vi "PH_BL-Master.contents.vi"   [LabVIEW 2014, in "PH_BL-Master.lvlib"]
doc: "This class is forseen to inspect the PHELIX beamline and to select the mode. Additional several settings can be chosen.\n\nThis class is part of the PHELIX user layer."
uses:
  PH_BL-Master.lvlib
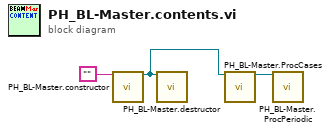
[diagram p0: block diagram]
diagram:
  n1 = call "PH_BL-Master.constructor.vi"("name"="") -> ("i ref out"=w1:refnum<vi>)  [unwired: 16 in, 2 out]
  n2 = call "PH_BL-Master.destructor.vi"("i ref in"=w1) -> ()  [unwired: 18 in, 1 out]
  n3 = call "PH_BL-Master.ProcCases.vi"("i ref in"=w1) -> ("i ref out"=w2:refnum<vi>)  [unwired: 16 in, 2 out]
  n4 = call "PH_BL-Master.ProcPeriodic.vi"("i ref in"=w2) -> ()  [unwired: 16 in, 3 out]
